vi "Start Discovery Service.vi"(8 "error in":errorcluster, 10 "cluster id":string, 11 "key file path":path) -> (0 "error out":errorcluster)   [LabVIEW 2020, in "Plug-In SDK Discovery V1 API.lvlib"]
doc: "This VI starts the MeasurementLink.DiscoveryService.exe."
uses:
  Plug-In SDK Discovery V1 API.lvlib
  <vilib>/Utility/sysdir.llb/System Directory Type.ctl
  Measurements/Helpers/Error Strings Global Internal.vi
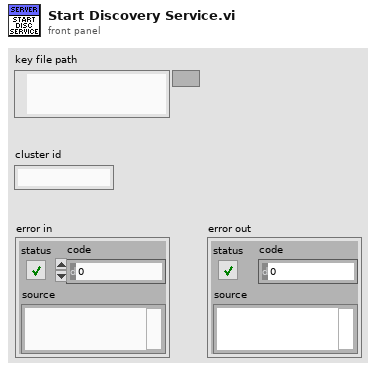
[diagram p1: front panel]
types:
  T1 = enum16{"open", "replace", "create", "open or create", "replace or create", "replace or create with confirmation"}
  T2 = typedef "System Directory Type.ctl" = i32
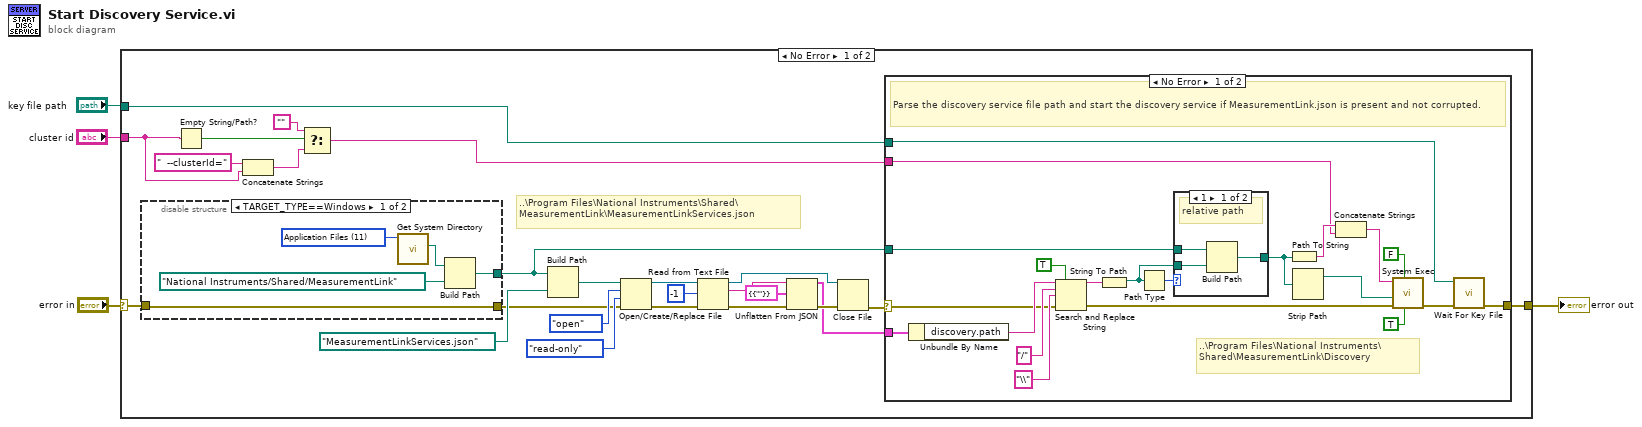
[diagram p0: block diagram]
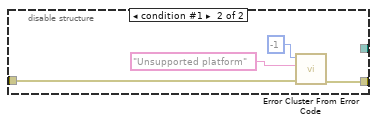
[diagram p2: hidden frame]
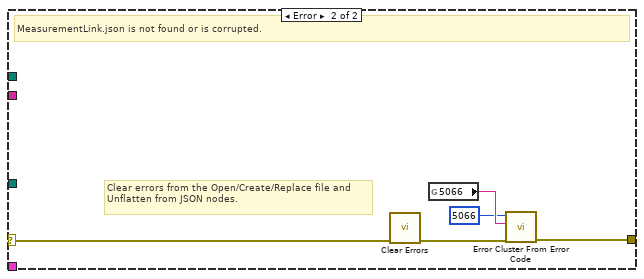
[diagram p4: hidden frame]
diagram:
  n1 = case shown="No Error" "error in" {
    selector: "error in" -> [w24 w69]
    tunnel: [w23 w69] -> w3
    tunnel: "key file path" -> [w22 _]
    tunnel: "cluster id" -> [w9 _]
    frame No Error {
      # "..\\Program Files\\National Instruments\\Shared\\MeasurementLink\\MeasurementLinkServices.json"
      n2 = disable-structure shown="TARGET_TYPE==Windows" {
        disable-tunnel: [w31 _] -> w21
        disable-tunnel: w24 -> [w30 w36]
        disable-tunnel: [w30 w35] -> w25
        frame condition #0 (active) {
          w34 = T2 11 items=["User Home"=0, "User Desktop"=1, "User Documents"=2, "User Application Data"=3, "User Preferences"=4, "User Temporary"=5, "Public Documents"=6, "Public Application Data"=7, "Public Preferences"=8, "Public Cache"=13, "System Core Libraries"=9, "System Installed Libraries"=10, "Application Files"=11, "Boot Volume Root"=12] ("system directory type")
          n3 = call <vilib>:"Get System Directory.vi"("system directory type"=w34) -> ("system directory"=w33:path)  [unwired: 10 in]
          n4 = Build Path(base path=w33, name or relative path=path "National Instruments/Shared/MeasurementLink") -> (appended path=w31:path)
        }
        frame condition #1 {
          n5 = call <vilib>:"Error Cluster From Error Code.vi"("error in (no error)"=w36, "error message (\"\")"="Unsupported platform" ("error message (\"\")"), "error code (0)"=-1) -> ("error out"=w35:errorcluster)  [unwired: 6 in]
        }
      }
      n6 = Empty String/Path?(string/path=w9) -> (empty?=w8:bool)
      n7 = Concatenate Strings("  --clusterId=" ("string"), w9) -> (w7:string)
      n8 = Select(t="", s=w8, f=w7) -> (s? t:f=w5:string)
      n9 = Build Path(base path=w21, name or relative path=path "MeasurementLinkServices.json") -> (appended path=w28:path)
      n10 = Open/Create/Replace File(file path (use dialog)=w28, error in=w25, operation (0:open)=T1."open", access (0:read/write)=enum16{"read/write", "read-only", "write-only"}."read-only") -> (refnum out=w13:refnum<file>, error out=w16:errorcluster)  [unwired: 2 in, 1 out]
      n11 = Read from Text File(file (use dialog)=w13, count=-1, error in=w16) -> (refnum out=w14:refnum<file>, text=w18:string, error out=w20:errorcluster)  [unwired: 1 in, 1 out]
      n12 = Unflatten From JSON(JSON string=w18, type and defaults=cluster{"discovery":cluster{"path":string}} {"discovery"={"path"=""}}, error in (no error)=w20) -> (value=w11:cluster{"discovery":cluster{"path":string}}, error out=w15:errorcluster)  [unwired: 4 in]
      n13 = Close File(refnum=w14, error in=w15) -> (error out=w12:errorcluster)  [unwired: 1 out]
      n14 = case shown="No Error" w12 {
        selector: w12 -> [w43 w68]
        tunnel: [w51 w66] -> w23
        tunnel: w22 -> [w50 _]
        tunnel: w21 -> [w46 _]
        tunnel: w11 -> [w42 _]
        tunnel: w5 -> [w39 _]
        frame No Error {
          # "..\\Program Files\\National Instruments\\Shared\\MeasurementLink\\Discovery"
          # "Parse the discovery service file path and start the discovery service if MeasurementLink.json is present and not corrupted."
          n15 = Unbundle By Name(w42) -> ("discovery.path"=w44:string)
          n16 = Search and Replace String(replace all?=TRUE ("replace all? (F)"), input string=w44, search string="/", replace string="\\" ("replace string (\"\")"), error in=w43) -> (result string=w47:string, error out=w56:errorcluster)  [unwired: 3 in, 2 out]
          n17 = String To Path(string=w47) -> (path=w48:path)
          n18 = Path Type(1:w48) -> (0:w49:i16)
          n19 = case shown="1" w49 {
            tunnel: [w62 w63] -> w45
            tunnel: w46 -> [w61 _]
            tunnel: w48 -> [w60 w63]
            frame 1 {
              # "relative path"
              n20 = Build Path(base path=w61, name or relative path=w60) -> (appended path=w62:path)
            }
            frame Default {
              # "absolute path"
            }
          }
          n21 = Path To String(path=w45) -> (string=w41:string)
          n22 = Strip Path(path=w45) -> (stripped path=w57:path)  [unwired: 1 out]
          n23 = Concatenate Strings(w41, w39) -> (w40:string)
          n24 = call <vilib>:"System Exec.vi"("run minimized? (F)"=TRUE, "wait until completion? (T)"=FALSE, "error in (no error)"=w56, "working directory"=w57, "command line"=w40) -> ("error out"=w53:errorcluster)  [unwired: 3 in, 3 out]
          n25 = call "Wait For Key File.vi"("error in"=w53, "key file path"=w50) -> ("error out"=w51:errorcluster)  [unwired: 9 in]
        }
        frame Error {
          # "Clear errors from the Open/Create/Replace file and Unflatten from JSON nodes."
          # "MeasurementLink.json is not found or is corrupted."
          n26 = call <vilib>:"Clear Errors.vi"("error in (no error)"=w68) -> ("error out"=w67:errorcluster)  [unwired: 5 in, 1 out]
          n27 = global read "Error Strings Global Internal.vi" "5066"() -> (w65:string)
          n28 = call <vilib>:"Error Cluster From Error Code.vi"("error in (no error)"=w67, "error message (\"\")"=w65, "error code (0)"=5066) -> ("error out"=w66:errorcluster)  [unwired: 6 in]
        }
      }
    }
    frame Error {
    }
  }
  "error out" <- w3
